vi "Registres à décalage.vi"() -> ()   [LabVIEW 2014]
panel:
  out "X(i-3)":i32
  out "X(i-2)":i32
  out "X(i-1)":i32
  out "X(i)":i32
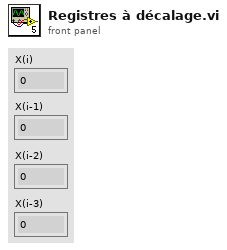
[diagram p1: front panel]
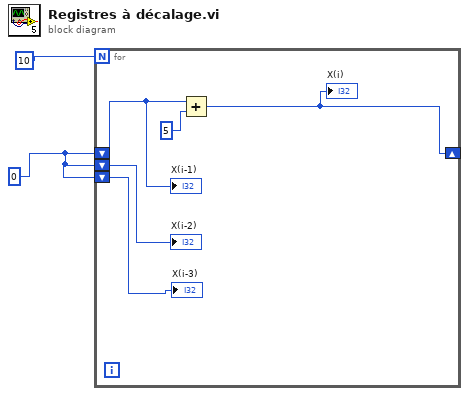
[diagram p0: block diagram]
diagram:
  w2 = 0
  n1 = for {
    N: 10 -> [_]
    shift-right: [w3] -> _
    shift-left: w2 -> [w5]
    shift-left: w2 -> [w6]
    shift-left: w2 -> [w7]
    n2 = Add(x=w5, y=5) -> (x+y=w3:i32)
    "X(i)" <- w3
    "X(i-1)" <- w5
    "X(i-2)" <- w6
    "X(i-3)" <- w7
  }
